vi "Listening Server - Close.vi"(8 "error in (no error)":errorcluster, 11 "Plugin in":refnum<class "Generic Plugin.lvclass">) -> (0 "error out":errorcluster, 3 "Plugin out":refnum<class "Generic Plugin.lvclass">)   [LabVIEW 2020, in "RxnRover.lvlib" / "Generic Plugin.lvclass"]
doc: "Closes the listening server VI reference and clears the corresponding class attribute."
uses:
  Generic Plugin.lvclass
  Generic Plugin.lvclass/Generic Plugin.ctl
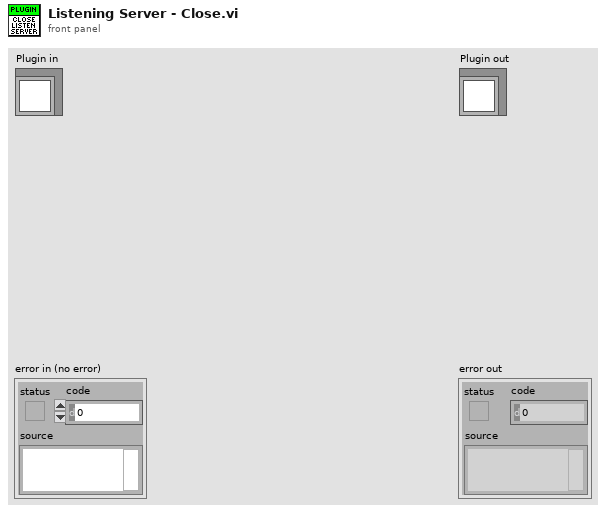
[diagram p1: front panel]
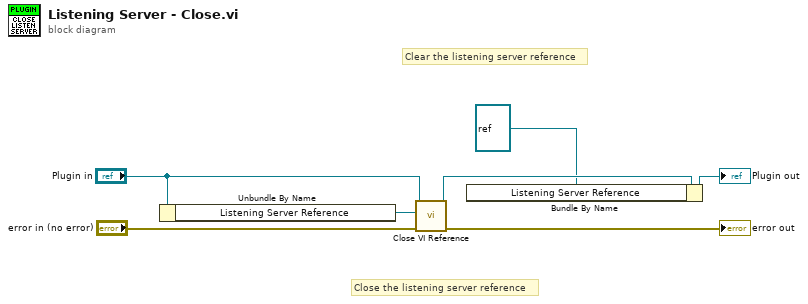
[diagram p0: block diagram]
diagram:
  # "Close the listening server reference"
  # "Clear the listening server reference"
  n1 = Unbundle By Name("Plugin in") -> ("Listening Server Reference"=w1:refnum<vi>)
  n2 = call "Close VI Reference.vi"("error in (no error)"="error in (no error)", "VI Refnum"=w1, "Plugin Server in"="Plugin in") -> ("error out"=→"error out":errorcluster, "Plugin Server out"=w7:refnum<class "Generic Plugin.lvclass">)  [unwired: 6 in, 1 out]
  n3 = Bundle By Name(cluster=w7, "Listening Server Reference"=refnum<vi> refnum ("Subpanel.Reference")) -> (→"Plugin out":refnum<class "Generic Plugin.lvclass">)
